vi "Close Notifiers.vi"(8 "error in":errorcluster) -> (0 "error out":errorcluster)   [LabVIEW 2017]
uses:
  Notifiers.ctl
panel:
  in  "Notifiers":T1
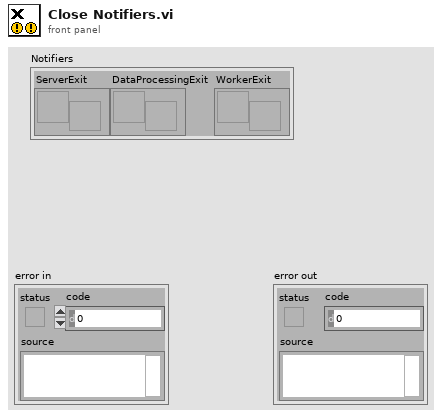
[diagram p1: front panel]
types:
  T1 = typedef "Notifiers.ctl" = cluster{"ServerExit":refnum<notifier>, "DataProcessingExit":refnum<notifier>, "WorkerExit":refnum<notifier>}
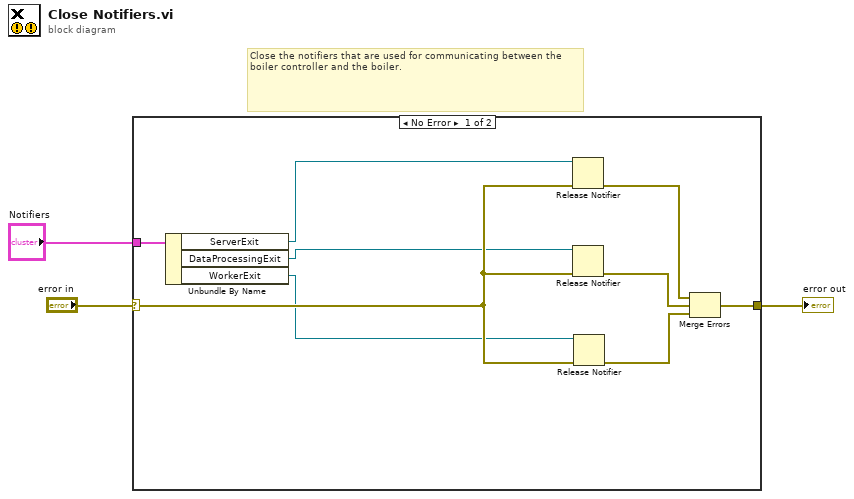
[diagram p0: block diagram]
diagram:
  # "Close the notifiers that are used for communicating between the boiler controller and the boiler."
  n1 = case shown="No Error" "error in" {
    selector: "error in" -> [w11 w13]
    tunnel: "Notifiers" -> [w7 _]
    tunnel: [w12 w13] -> w2
    frame No Error {
      n2 = Unbundle By Name(w7) -> ("ServerExit"=w6:refnum<notifier>, "DataProcessingExit"=w5:refnum<notifier>, "WorkerExit"=w4:refnum<notifier>)
      n3 = Release Notifier(notifier=w6, error in (no error)=w11) -> (error out=w8:errorcluster)  [unwired: 1 in, 2 out]
      n4 = Release Notifier(notifier=w5, error in (no error)=w11) -> (error out=w9:errorcluster)  [unwired: 1 in, 2 out]
      n5 = Release Notifier(notifier=w4, error in (no error)=w11) -> (error out=w10:errorcluster)  [unwired: 1 in, 2 out]
      n6 = Merge Errors(w8, w9, w10) -> (w12:errorcluster)
    }
    frame Error {
    }
  }
  "error out" <- w2
